vi "WriteTemperature.vi"(8 "error in (no error)":errorcluster, 10 "Temperature":dbl, 11 "AirCondition in":refnum<class "AirCondition.lvclass">) -> (0 "error out":errorcluster, 3 "AirCondition out":refnum<class "AirCondition.lvclass">)   [LabVIEW 2013, in "AirCondition.lvclass"]
uses:
  AirCondition.lvclass
  AirCondition.lvclass/AirCondition.ctl
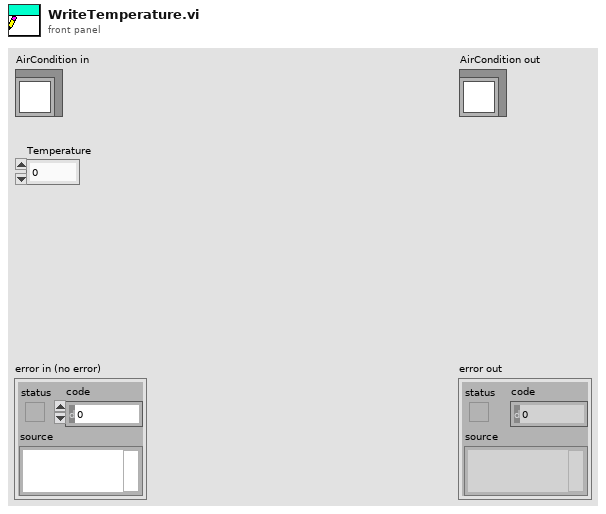
[diagram p1: front panel]
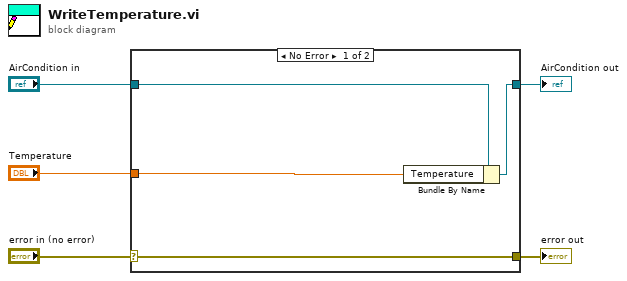
[diagram p0: block diagram]
diagram:
  n1 = case shown="No Error" "error in (no error)" {
    selector: "error in (no error)" -> [w9 w10]
    tunnel: [w9 w10] -> w4
    tunnel: [w7 w11] -> w2
    tunnel: "AirCondition in" -> [w8 w11]
    tunnel: "Temperature" -> [w6 _]
    frame No Error {
      n2 = Bundle By Name(cluster=w8, "Temperature"=w6) -> (w7:refnum<class "AirCondition.lvclass">)
    }
    frame Error {
    }
  }
  "error out" <- w4
  "AirCondition out" <- w2
